vi "MQTT_Publish.vi"(6 "Message ID":u16=10 format="%x", 7 "Publish Meta":cluster{"QoS":T1, "Retain":T2, "DUP":T3}, 8 "error in (no error)":errorcluster, 9 "Message to be published":string=" Message", 10 "Topic":string="a/b", 11 "connection ID":refnum<k5>) -> (0 "error out":errorcluster, 3 "connection ID out":refnum<k5>)   [LabVIEW 2013, in "MQTT_Functions.lvlib"]
doc: "This VI publishes a message to a registered topic.\n\n© 2015 - daq.io, LLC - Peter Adelhardt"
uses:
  MQTT_Functions.lvlib
  Controls/MessageType.ctl
  Controls/QoS.ctl
  Controls/Retain_Flag.ctl
  Controls/DUP_Flag.ctl
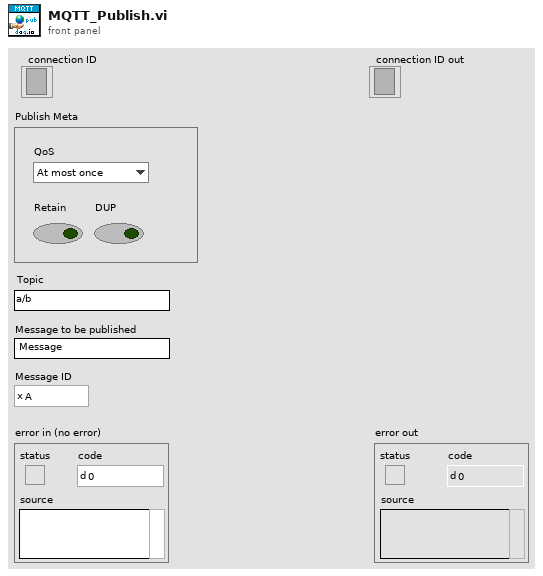
[diagram p1: front panel]
types:
  T1 = typedef "MQTT_Functions.lvlib/QoS.ctl" = enum8{"At most once", "At least once", "Exactly once", "Reserved"}
  T2 = typedef "MQTT_Functions.lvlib/Retain_Flag.ctl" = bool
  T3 = typedef "MQTT_Functions.lvlib/DUP_Flag.ctl" = bool
  T4 = typedef "MQTT_Functions.lvlib/MessageType.ctl" = enum32{"Reserved", "CONNECT", "CONNACK", "PUBLISH", "PUBACK", "PUBREC", "PUBREL", "PUBCOMP", "SUBSCRIBE", "SUBACK", "UNSUBSCRIBE", "UNSUBACK", "PINGREQ", "PINGRESP", "DISCONNECT", "Reserved2"}
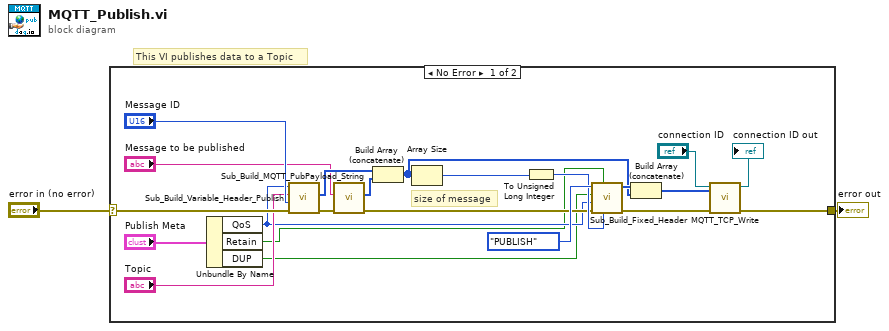
[diagram p0: block diagram]
diagram:
  # "This VI publishes data to a Topic"
  n1 = case shown="No Error" "error in (no error)" {
    selector: "error in (no error)" -> [w23 w25]
    tunnel: [w5 w25] -> w1
    frame No Error {
      # "size of message"
      n2 = Unbundle By Name("Publish Meta") -> ("QoS"=w10:T1, "Retain"=w9:T2, "DUP"=w8:T3)
      n3 = call "Sub_Build_Variable_Header_Publish.vi"("error in (no error)"=w23, "Message ID"="Message ID", "Topic Name"="Topic", "QoS"=w10) -> ("error out"=w19:errorcluster, "Variable Header"=w17:u8[])  [unwired: 6 in]
      n4 = call "Sub_Build_MQTT_PubPayload_String.vi"("error in (no error)"=w19, "String to be encoded"="Message to be published") -> ("error out"=w18:errorcluster, "UTF8 Byte Array"=w16:u8[])  [unwired: 8 in]
      n5 = Build Array (concatenate)(w17, w16) -> (w14:u8[])
      n6 = Array Size(array=w14) -> (size(s)=w20:i32)
      n7 = To Unsigned Long Integer(number=w20) -> (unsigned 32bit integer=w21:u32)
      n8 = call "Sub_Build_Fixed_Header.vi"("Remaining Length"=w21, "Retain"=w9, "error in (no error)"=w18, "QoS"=w10, "DUP"=w8, "MessageType"=MessageType."PUBLISH") -> ("error out"=w7:errorcluster, "Fixed Header"=w15:u8[])  [unwired: 4 in]
      n9 = Build Array (concatenate)(w15, w14) -> (w6:u8[])
      n10 = call "MQTT_TCP_Write.vi"("error in (no error)"=w7, "data in"=w6, "connection ID"="connection ID") -> ("error out"=w5:errorcluster, "connection ID out"=→"connection ID out":refnum<k5>)  [unwired: 6 in, 1 out]
    }
    frame Error {
    }
  }
  "error out" <- w1
